vi "test_TCP_TCP Clear Error.vi"(8 "error in (no error)":errorcluster, 11 "TestCase in":refnum<class "Ethernet Protocol Tests.lvclass">) -> (0 "error out":errorcluster, 3 "TestCase out":refnum<class "Ethernet Protocol Tests.lvclass">)   [LabVIEW 2019, in "Ethernet Protocol Tests.lvclass"]
uses:
  Ethernet Protocol Tests.lvclass
  ListenerVi/Listener.lvclass
  TCP/TCP.lvclass
  D:/GitRepository/niveristand-instrument-addon-classes/Source/Protocols/Protocol Parent/Protocol Parent.lvclass
  ListenerVi/ListenerClassControls/Operation Ctl.ctl
  TCP/TCP.lvclass/TCP.ctl
  Protocol Parent/Methods/Read Parameter.ctl
  <vilib>/addons/_JKI Toolkits/VI Tester/TestCase.llb/TestCase.lvclass
  Protocol Parent/Protocol Parent.lvclass
  C:/Program Files (x86)/National Instruments/LabVIEW 2019/vi.lib/addons/_JKI Toolkits/VI Tester/TestCase.llb/TestCase.lvclass
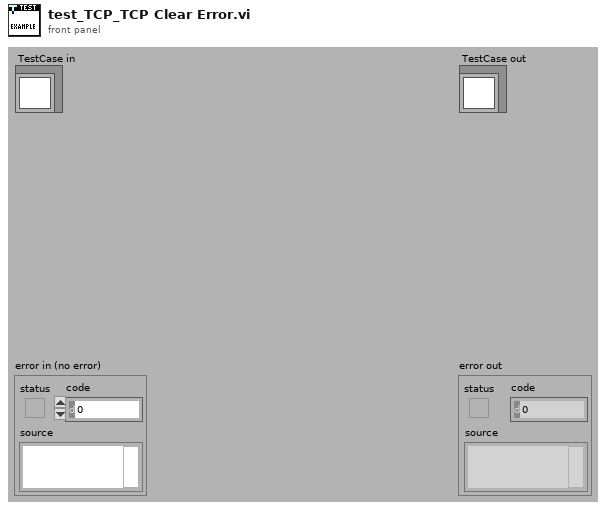
[diagram p1: front panel]
types:
  T1 = typedef "Protocols.lvlib/Protocol Parent.lvclass/Read Parameter.ctl" = cluster{"Wait Type":enum16{"Byte Count", "Wait sec"}, "Wait Value":dbl}
  T2 = typedef "Operation Ctl.ctl" = enum16{"Read", "Write"}
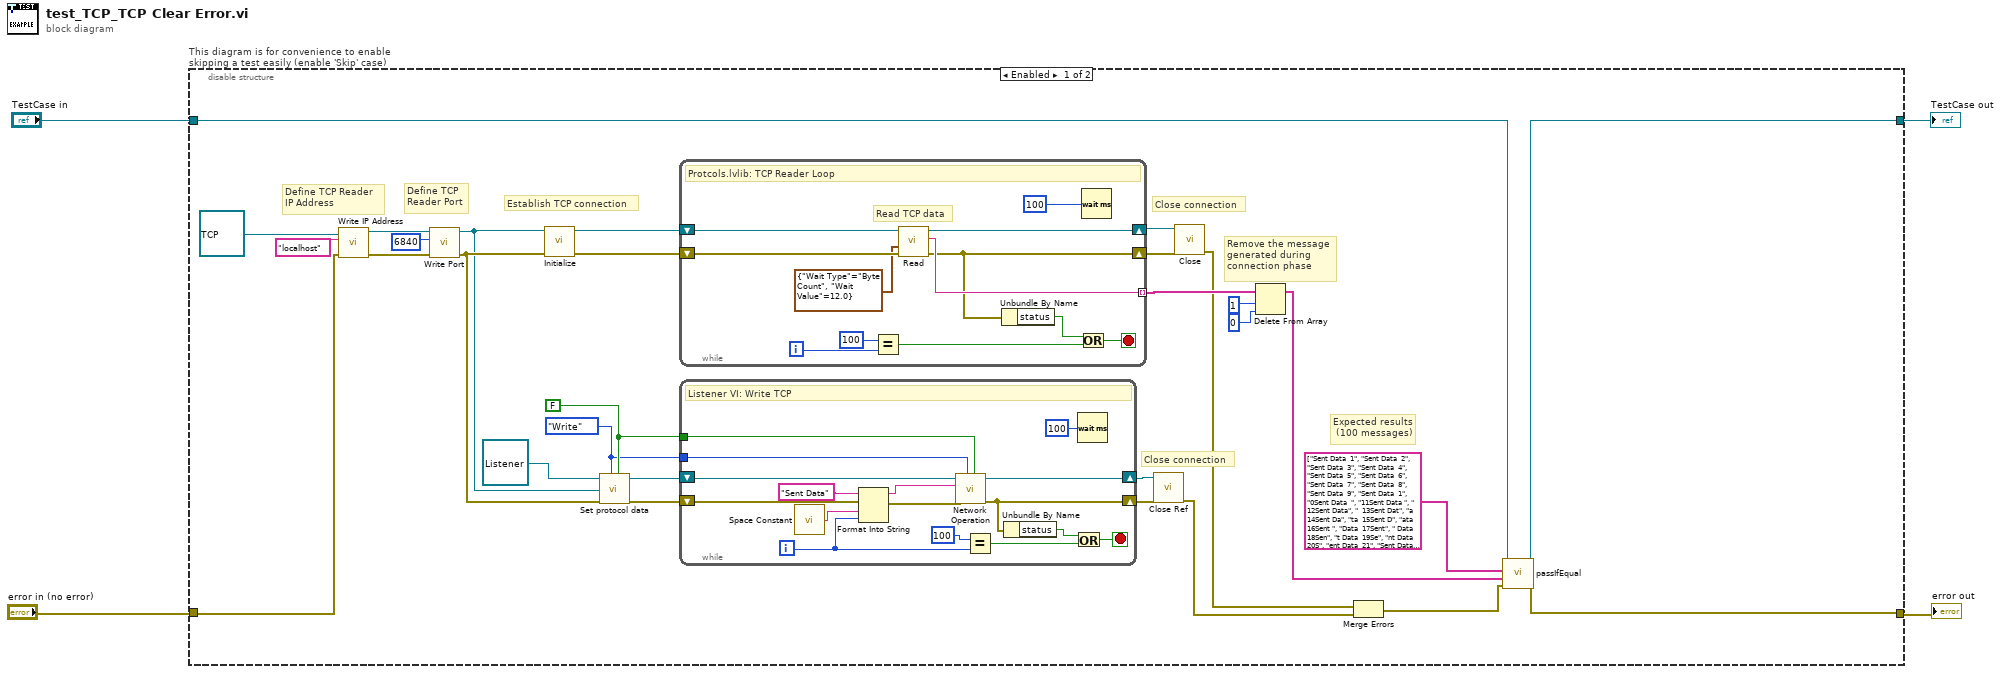
[diagram p0: block diagram]
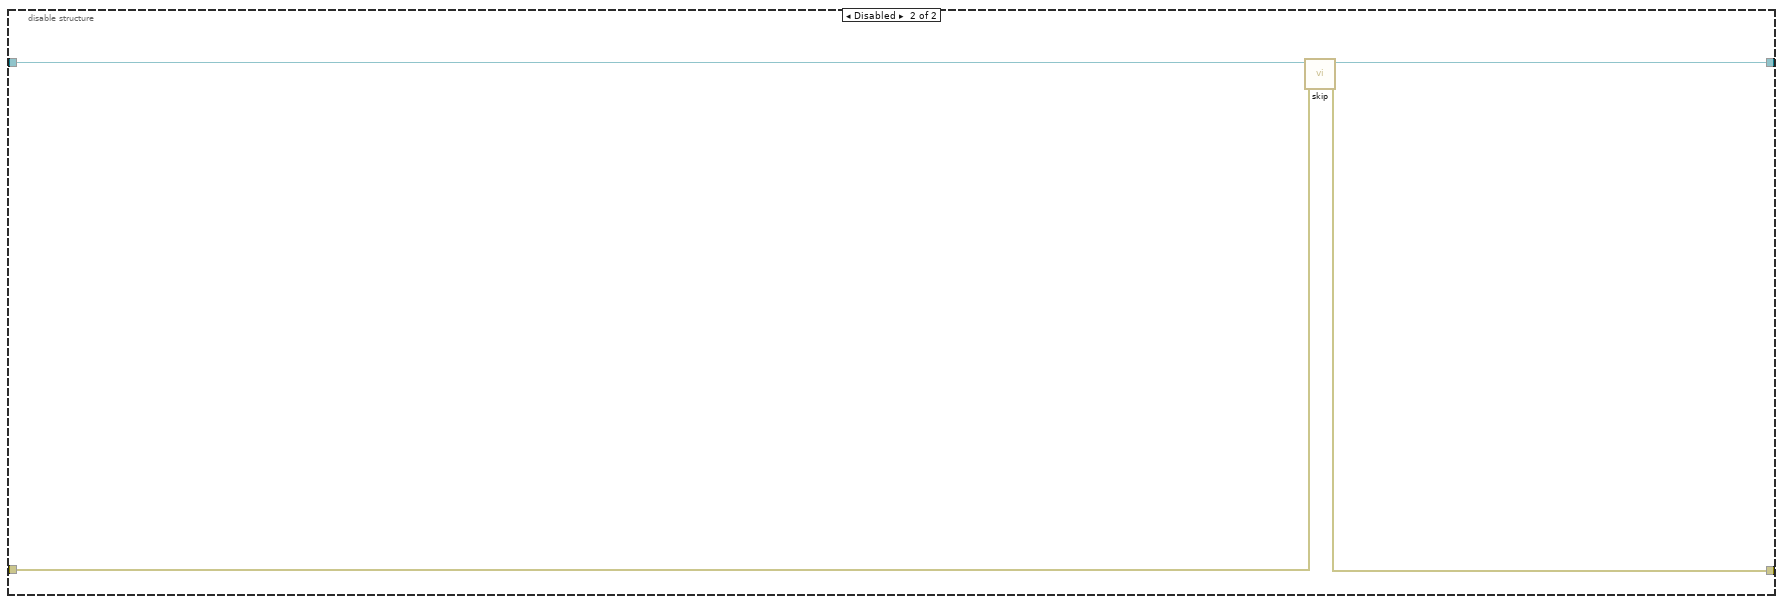
[diagram p2: hidden frame]
diagram:
  n1 = disable-structure "This diagram is for convenience to enable skipping a test easily (enable 'Skip' case)" shown="Enabled" {
    disable-tunnel: "TestCase in" -> [w34 w66]
    disable-tunnel: [w33 w64] -> w1
    disable-tunnel: [w32 w65] -> w3
    disable-tunnel: "error in (no error)" -> [w27 w63]
    frame Enabled {
      w10 = Operation_Ctl."Write" ("Operation")
      w11 = FALSE ("AK?")
      # "Establish TCP connection"
      # "Close connection"
      # "Close connection"
      # "Remove the message\ngenerated during \nconnection phase"
      # "Expected results\n (100 messages)"
      # "Define TCP \nReader Port"
      # "Define TCP Reader \nIP Address"
      n2 = call "Write IP Address.vi"("error in (no error)"=w27, "IP Address"="localhost", "Ethernet in"=refnum<class "TCP.lvclass"> refnum ("Protocols.lvlib:TCP.lvclass")) -> ("error out"=w29:errorcluster, "Ethernet out"=w30:refnum<class "TCP.lvclass">)  [unwired: 7 in]
      n3 = call "Write Port.vi"("error in (no error)"=w29, "Port"=u16 6840, "Ethernet in"=w30) -> ("error out"=w9:errorcluster, "Ethernet out"=w6:refnum<class "TCP.lvclass">)  [unwired: 7 in]
      n4 = call-dynamic "Initialize.vi"("error in (no error)"=w9, "Ethernet in"=w6) -> ("error out"=w8:errorcluster, "Ethernet out"=w7:refnum<class "TCP.lvclass">)  [unwired: 8 in]
      n5 = call "Set protocol data.vi"("AK?"=w11, "Operation"=w10, "error in (no error)"=w9, "Protocols.lvlib:Protocol Parent.lvclass"=w6, "Listener In.lvclass"=refnum<class "Listener.lvclass"> refnum ("Listener.lvclass")) -> ("error out"=w13:errorcluster, "Listener Out.lvclass"=w12:refnum<class "Listener.lvclass">)  [unwired: 5 in]
      n6 = while {
        shift-right: [w56] -> w21
        shift-left: w8 -> [w61]
        shift-right: [w60] -> w20
        shift-left: w7 -> [w62]
        tunnel: [w59] -> w25 mode=indexing
        i -> [w58]
        stop <- w53 stop-if-true
        # "Read TCP data"
        # "Protcols.lvlib: TCP Reader Loop"
        n7 = Equal?(x=100, y=w58) -> (x = y?=w54:bool)
        n8 = call-dynamic "Read.vi"("error in (no error)"=w61, "Variant"=T1 {"Wait Type"=enum."Byte Count", "Wait Value"=12.0} ("Read Parameter"), "Ethernet in"=w62) -> ("error out"=w56:errorcluster, "String"=w59:string, "Ethernet out"=w60:refnum<class "TCP.lvclass">)  [unwired: 6 in]
        n9 = Unbundle By Name(w56) -> ("status"=w55:bool)
        n10 = Or(x=w55, y=w54) -> (x .or. y?=w53:bool)
        n11 = Wait (ms)(milliseconds to wait=u32 100) -> ()  [unwired: 1 out]
      }
      n12 = while {
        shift-right: [w46] -> w17
        shift-left: w13 -> [w37]
        shift-right: [w45] -> w18
        shift-left: w12 -> [w38]
        tunnel: w11 -> [w36]
        tunnel: w10 -> [w35]
        i -> [w41]
        stop <- w49 stop-if-true
        # "Listener VI: Write TCP"
        n13 = call <vilib>:"Space Constant.vi"() -> ("String"=w42:string)
        n14 = Format Into String(initial string="Sent Data", error in=w37, w42, w41) -> (resulting string=w40:string, error out=w39:errorcluster)  [unwired: 1 in]
        n15 = call "Network Operation.vi"("AK?"=w36, "Operation"=w35, "error in (no error)"=w39, "Message"=w40, "Listener In.lvclass"=w38) -> ("error out"=w46:errorcluster, "Listener Out.lvclass"=w45:refnum<class "Listener.lvclass">)  [unwired: 5 in]
        n16 = Equal?(x=100, y=w41) -> (x = y?=w47:bool)
        n17 = Unbundle By Name(w46) -> ("status"=w50:bool)
        n18 = Or(x=w50, y=w47) -> (x .or. y?=w49:bool)
        n19 = Wait (ms)(milliseconds to wait=u32 100) -> ()  [unwired: 1 out]
      }
      n20 = call "Close Ref.vi"("error in (no error)"=w17, "Listener In.lvclass"=w18) -> ("error out"=w16:errorcluster)  [unwired: 9 in]
      n21 = call-dynamic "Close.vi"("error in (no error)"=w21, "Ethernet in"=w20) -> ("error out"=w19:errorcluster)  [unwired: 8 in, 1 out]
      n22 = Delete From Array(array=w25, length=1 ("index"), index=0 ("length")) -> (array with subset deleted=w22:string[])  [unwired: 1 out]
      n23 = Merge Errors(w19, w16) -> (w26:errorcluster)
      n24 = call-dynamic "passIfEqual.vi"("error in (no error)"=w26, "y"=w22, "x"=string[] ["Sent Data  1", "Sent Data  2", "Sent Data  3", "Sent Data  4", "Sent Data  5", "Sent Data  6", "Sent Data  7", "Sent Data  8", "Sent Data  9", "Sent Data  1", "0Sent Data  ", "11Sent Data ", " 12Sent Data", "  13Sent Dat", "a  14Sent Da", "ta  15Sent D", "ata  16Sent ", "Data  17Sent", " Data  18Sen", "t Data  19Se", "nt Data  20S", "ent Data  21", "Sent Data  2", "2Sent Data  ", "23Sent Data ", " 24Sent Data", "  25Sent Dat", "a  26Sent Da", "ta  27Sent D", "ata  28Sent ", "Data  29Sent", " Data  30Sen", "t Data  31Se", "nt Data  32S", "ent Data  33", "Sent Data  3", "4Sent Data  ", "35Sent Data ", " 36Sent Data", "  37Sent Dat", "a  38Sent Da", "ta  39Sent D", "ata  40Sent ", "Data  41Sent", " Data  42Sen", "t Data  43Se", "nt Data  44S", "ent Data  45", "Sent Data  4", "6Sent Data  ", "47Sent Data ", " 48Sent Data", "  49Sent Dat", "a  50Sent Da", "ta  51Sent D", "ata  52Sent ", "Data  53Sent", " Data  54Sen", "t Data  55Se", "nt Data  56S", "ent Data  57", "Sent Data  5", "8Sent Data  ", "59Sent Data ", " 60Sent Data", "  61Sent Dat", "a  62Sent Da", "ta  63Sent D", "ata  64Sent ", "Data  65Sent", " Data  66Sen", "t Data  67Se", "nt Data  68S", "ent Data  69", "Sent Data  7", "0Sent Data  ", "71Sent Data ", " 72Sent Data", "  73Sent Dat", "a  74Sent Da", "ta  75Sent D", "ata  76Sent ", "Data  77Sent", " Data  78Sen", "t Data  79Se", "nt Data  80S", "ent Data  81", "Sent Data  8", "2Sent Data  ", "83Sent Data ", " 84Sent Data", "  85Sent Dat", "a  86Sent Da", "ta  87Sent D", "ata  88Sent ", "Data  89Sent", " Data  90Sen", "t Data  91Se", "nt Data  92S", "ent Data  93"] ("array w/ subset deleted"), "TestCase in"=w34) -> ("error out"=w32:errorcluster, "TestCase out"=w33:refnum<class "Ethernet Protocol Tests.lvclass">)  [unwired: 6 in]
    }
    frame Disabled {
      # "skip test result while test is under development"
      n25 = call <vilib>:"skip.vi"("error in (no error)"=w63, "TestCase in"=w66) -> ("error out"=w65:errorcluster, "TestCase out"=w64:refnum<class "Ethernet Protocol Tests.lvclass">)  [unwired: 8 in]
    }
  }
  "error out" <- w3
  "TestCase out" <- w1
